vi "AcquireSinglePointData.vi"(8 "error in (no error)":errorcluster, 9 "Numeric":i32, 11 "Channel":T1={"Name"="", "Hardware Channel"="", "ChannelType"="", "TrendPoint Id"="", "Value"=0.0, "Slope"=0.0, "Offset"=0.0, "IO variable"="", "datatype"=enum."Boolean", "Properties"=[]}) -> (0 "error out":errorcluster, 1 "Value":dbl, 2 "Status":string)   [LabVIEW 2017, in "ScanEngine.lvlib"]
uses:
  <vilib>/addons/InsightCM/Devices/Shared/Common/ScanEngine/ScanEngine.lvlib
  <vilib>/addons/InsightCM/Devices/Shared/Common/ScanEngine/controls/Channel.ctl
  <vilib>/Utility/Data Type/Type Definitions/Data Type.ctl
  <vilib>/addons/InsightCM/MessageBus/Base/controls/KeyValuePair.ctl
  <vilib>/addons/InsightCM/Utilities/ChannelStatus/ChannelStatus.lvlib
  <vilib>/Utility/Data Type/NI_Data Type.lvlib
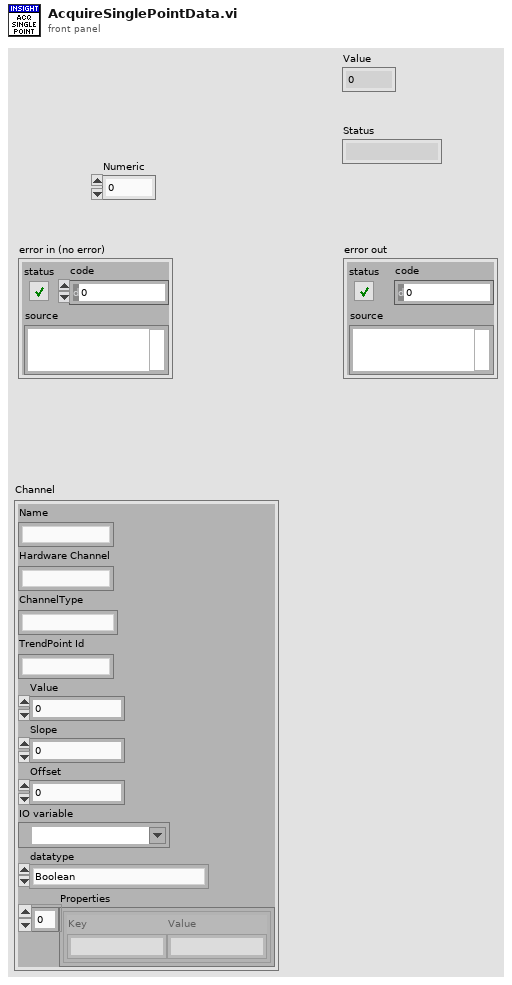
[diagram p1: front panel]
types:
  T1 = typedef "ScanEngine.lvlib/Channel.ctl" = cluster{"Name":string, "Hardware Channel":string, "ChannelType":string, "TrendPoint Id":string, "Value":sgl, "Slope":dbl, "Offset":dbl, "IO variable":refnum<k21>, "datatype":T2, "Properties":T3[]}
  T2 = typedef "NI_Data Type.lvlib/Data Type.ctl" = enum8{"Invalid Type", "Void", "I8", "I16", "I32", "I64", "U8", "U16", "U32", "U64", "Single Float", "Double Float", "Extended Float", "Single Complex", "Double Complex", "Extended Complex", "Enum U8", "Enum U16", "Enum U32", "Enum U64", "Single Float With Unit", "Double Float With Unit", "Extended Float With Unit", "Single Complex with Unit", "Double Complex with Unit", "Extended Complex with Unit", "Boolean", "String", "Path", "Picture", "Tag", "Array", "Cluster", "Variant", "LV Variant", "Waveform", "Timestamp", "Digital Waveform", "Digital Data", "ExpressData", "Refnum", "External Data", "VI", "Poly VI", "LabVIEW Class Instance", "Fixed Point"}
  T3 = typedef "KeyValuePair.ctl" = cluster{"Key":string, "Value":string}
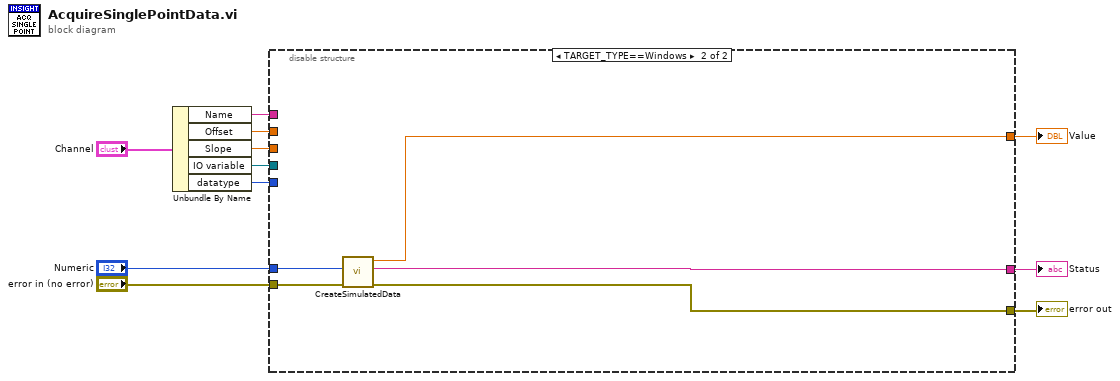
[diagram p0: block diagram]
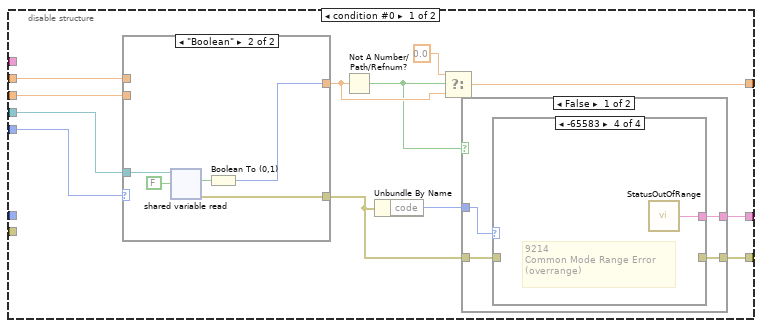
[diagram p2: hidden frame]
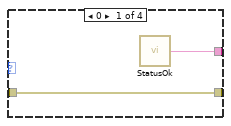
[diagram p3: hidden frame]
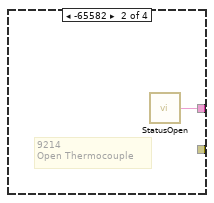
[diagram p4: hidden frame]
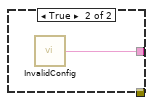
[diagram p6: hidden frame]
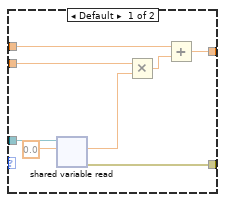
[diagram p7: hidden frame]
diagram:
  n1 = Unbundle By Name("Channel") -> ("Name"=w1:string, "Offset"=w2:dbl, "Slope"=w3:dbl, "IO variable"=w5:refnum<k21>, "datatype"=w4:T2)
  n2 = disable-structure shown="TARGET_TYPE==Windows" {
    disable-tunnel: w4 -> [w23 _]
    disable-tunnel: w5 -> [w22 _]
    disable-tunnel: [w13 w51] -> w6
    disable-tunnel: "error in (no error)" -> [_ w50]
    disable-tunnel: [w19 w48] -> w9
    disable-tunnel: "Numeric" -> [_ w49]
    disable-tunnel: [w18 w47] -> w10
    disable-tunnel: w3 -> [w17 _]
    disable-tunnel: w2 -> [w16 _]
    disable-tunnel: w1 -> [_ _]
    frame condition #0 {
      n3 = case shown="\"Boolean\"" w23 {
        tunnel: [w41 w46] -> w21
        tunnel: [w34 w43] -> w14
        tunnel: w22 -> [w39 w42]
        tunnel: w17 -> [w37 _]
        tunnel: w16 -> [w35 _]
        frame Default {
          n4 = shared-variable-read(w39, 0.0) -> (w41:errorcluster, w38:dbl)  [unwired: 1 in, 2 out]
          n5 = Multiply(x=w37, y=w38) -> (x*y=w36:dbl)
          n6 = Add(x=w35, y=w36) -> (x+y=w34:dbl)
        }
        frame "Boolean" {
          n7 = shared-variable-read(w42, FALSE) -> (w46:errorcluster, w44:bool)  [unwired: 1 in, 2 out]
          n8 = Boolean To (0,1)(Boolean=w44) -> (0, 1=w43:i16)
        }
      }
      n9 = Not A Number/Path/Refnum?(number/path/refnum=w14) -> (NaN/Path/Refnum?=w12:bool)
      n10 = Unbundle By Name(w21) -> ("code"=w20:i32)
      n11 = Select(t=0.0 ("Value"), s=w12, f=w14) -> (s? t:f=w13:dbl)
      n12 = case shown="False" w12 {
        tunnel: w21 -> [w27 _]
        tunnel: w20 -> [w26 _]
        tunnel: [w25 _] -> w19
        tunnel: [w24 w33] -> w18
        frame False {
          n13 = case shown="-65583" w26 {
            tunnel: w27 -> [w29 _ w31 _]
            tunnel: [w29 _ w31 _] -> w25
            tunnel: [w28 w30 _ w32] -> w24
            frame 0 {
              n14 = call <vilib>:"StatusOk.vi"() -> ("status"=w28:string)  [unwired: 5 in]
            }
            frame -65582 {
              # "9214\nOpen Thermocouple"
              n15 = call <vilib>:"StatusOpen.vi"() -> ("status"=w30:string)  [unwired: 5 in]
            }
            frame Default {
              # "unknown error, pass through"
            }
            frame -65583 {
              # "9214\nCommon Mode Range Error\n(overrange)"
              n16 = call <vilib>:"StatusOutOfRange.vi"() -> ("status"=w32:string)  [unwired: 5 in]
            }
          }
        }
        frame True {
          n17 = call <vilib>:"InvalidConfig.vi"() -> ("status"=w33:string)  [unwired: 5 in]
        }
      }
    }
    frame condition #1 (active) {
      n18 = call <vilib>:"CreateSimulatedData.vi"("error in (no error)"=w50, "index"=w49) -> ("error out"=w48:errorcluster, "channel status"=w47:string, "value"=w51:dbl)  [unwired: 7 in]
    }
  }
  "Status" <- w10
  "error out" <- w9
  "Value" <- w6
